vi "FTDI SPI BASE AB-Set.vi"(4 "nCS":u8 max=4 step=1, 5 "ClockRate":u32=50000, 6 "Set Out-B (0-7)":bool[](array[boolean]), 7 "Set Out-A (0-7)":bool[](array[boolean]), 8 "Use Extra":bool, 9 "Set Channel":u16(ring) items=["Ch-A", "Ch-B"], 10 "Addr":T1 items=["Addr-0", "Addr-1", "Addr-2", "Addr-3", "Addr-4", "Addr-5", "Addr-6", "Addr-7"], 11 "Handler In":u32) -> (0 "error out":errorcluster, 2 "Latch Reg":u32 format="%b", 3 "Handler Out":u32)   [LabVIEW 2018]
uses:
  PROJEKT/NIKO/Labview/Niko V4/FTDI SPI/Ctl/Sub Addr.ctl
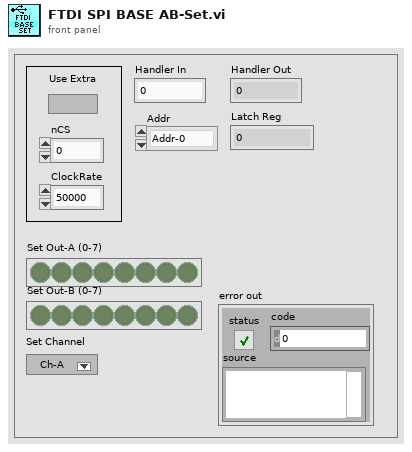
[diagram p1: front panel]
types:
  T1 = typedef "Sub Addr.ctl" = u16
  T2 = cluster{"ClockRate":u32, "LatencyTimer":u8, "configOptions 24-31":i8, "configOptions 16-23":i8, "configOptions 8-15":i8, "configOptions 0-7":u32, "Pin":u32, "reserved":u16}
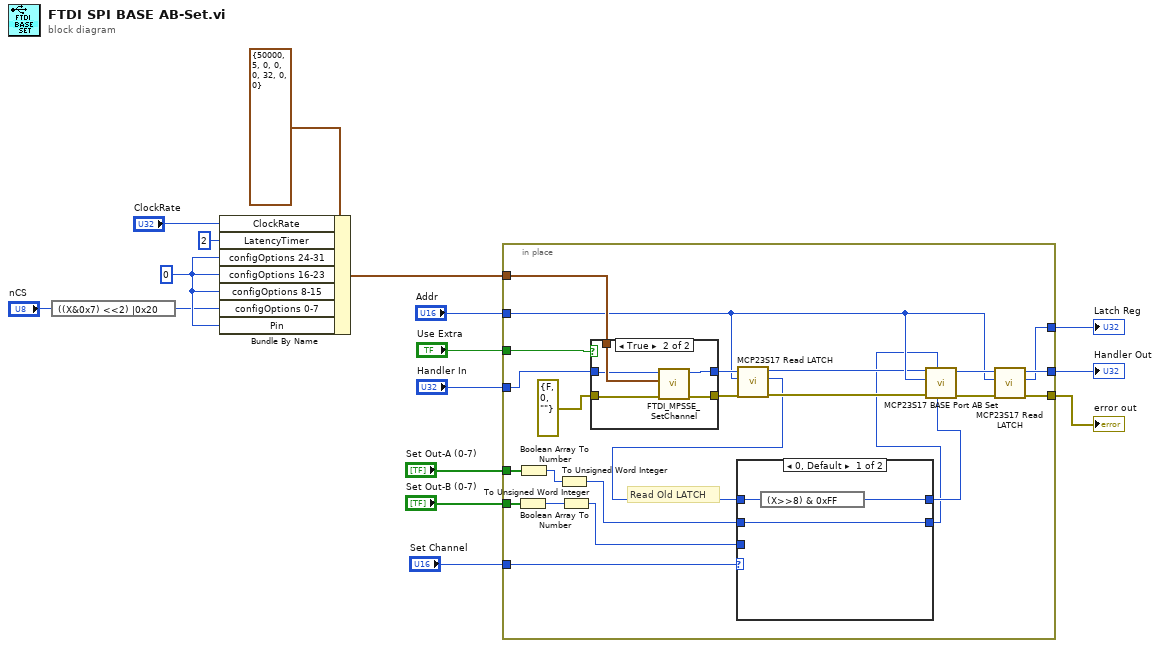
[diagram p0: block diagram]
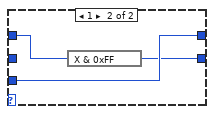
[diagram p2: hidden frame]
diagram:
  w12 = i8 0 ("configOptions 16-23")
  n1 = expression code="((X&0x7) <<2) |0x20"("nCS") -> (w10:u8)
  n2 = Bundle By Name(cluster=T2 {"ClockRate"=50000, "LatencyTimer"=5, "configOptions 24-31"=0, "configOptions 16-23"=0, "configOptions 8-15"=0, "configOptions 0-7"=32, "Pin"=0, "reserved"=0} ("config"), "ClockRate"="ClockRate", "LatencyTimer"=u8 2, "configOptions 24-31"=w12, "configOptions 16-23"=w12, "configOptions 8-15"=w12, "configOptions 0-7"=w10, "Pin"=w12) -> (w8:T2)
  n3 = in-place {
    in-place-border: "Handler In" -> [w40]
    in-place-border: "Addr" -> [w27]
    in-place-border: w8 -> [w38]
    in-place-border: [w32] -> w7
    in-place-border: [w34] -> w6
    in-place-border: "Use Extra" -> [w37]
    in-place-border: "Set Out-A (0-7)" -> [w36]
    in-place-border: "Set Out-B (0-7)" -> [w31]
    in-place-border: [w30] -> w2
    in-place-border: "Set Channel" -> [w24]
    # "Read Old LATCH"
    n4 = Boolean Array To Number(Boolean array=w31) -> (number=w23:u32)
    n5 = Boolean Array To Number(Boolean array=w36) -> (number=w22:u32)
    n6 = To Unsigned Word Integer(number=w22) -> (unsigned 16bit integer=w20:u16)
    n7 = To Unsigned Word Integer(number=w23) -> (unsigned 16bit integer=w21:u16)
    n8 = case shown="True" w37 {
      tunnel: w40 -> [w48 w49]
      tunnel: [w48 w52] -> w28
      tunnel: [w47 w53] -> w29
      tunnel: errorcluster {"status"=FALSE, "code"=0, "source"=""} ("error constant") -> [w47 w50]
      tunnel: w38 -> [_ w51]
      frame False {
      }
      frame True {
        n9 = call "FTDI_MPSSE_SetChannel.vi"("error in (no error)"=w50, "config"=w51, "handle"=w49) -> ("error out"=w53:errorcluster, "handle out"=w52:u32)  [unwired: 7 in]
      }
    }
    n10 = call "MCP23S17 Read LATCH.vi"("error in (no error)"=w29, "Addr"=w27, "handle"=w28) -> ("error out"=w25:errorcluster, "LATCH"=w19:u16, "handle out"=w26:u32)  [unwired: 4 in, 2 out]
    n11 = case shown="0, Default" w24 {
      tunnel: w21 -> [_ w46]
      tunnel: w20 -> [w41 _]
      tunnel: w19 -> [w43 w45]
      tunnel: [w42 w46] -> w18
      tunnel: [w41 w44] -> w17
      frame 0, Default {
        n12 = expression code="(X>>8) & 0xFF"(w43) -> (w42:u16)
      }
      frame 1 {
        n13 = expression code="X & 0xFF"(w45) -> (w44:u16)
      }
    }
    n14 = call "MCP23S17 BASE Port AB Set.vi"("Ch-B"=w18, "Ch-A"=w17, "error in (no error)"=w25, "Addr"=w27, "handle"=w26) -> ("error out"=w35:errorcluster, "handle out"=w33:u32)  [unwired: 5 in]
    n15 = call "MCP23S17 Read LATCH.vi"("error in (no error)"=w35, "Addr"=w27, "handle"=w33) -> ("error out"=w34:errorcluster, "LATCH"=w30:u16, "handle out"=w32:u32)  [unwired: 4 in, 2 out]
  }
  "Handler Out" <- w7
  "error out" <- w6
  "Latch Reg" <- w2
